vi "DataLogging.vi"() -> ()   [LabVIEW 2016]
uses:
  <vilib>/Utility/file.llb/Write Delimited Spreadsheet (string).vi
  <vilib>/Utility/file.llb/Write Delimited Spreadsheet (DBL).vi
panel:
  out "Elapsed Time":dbl
  in  "stop":bool
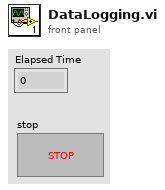
[diagram p1: front panel]
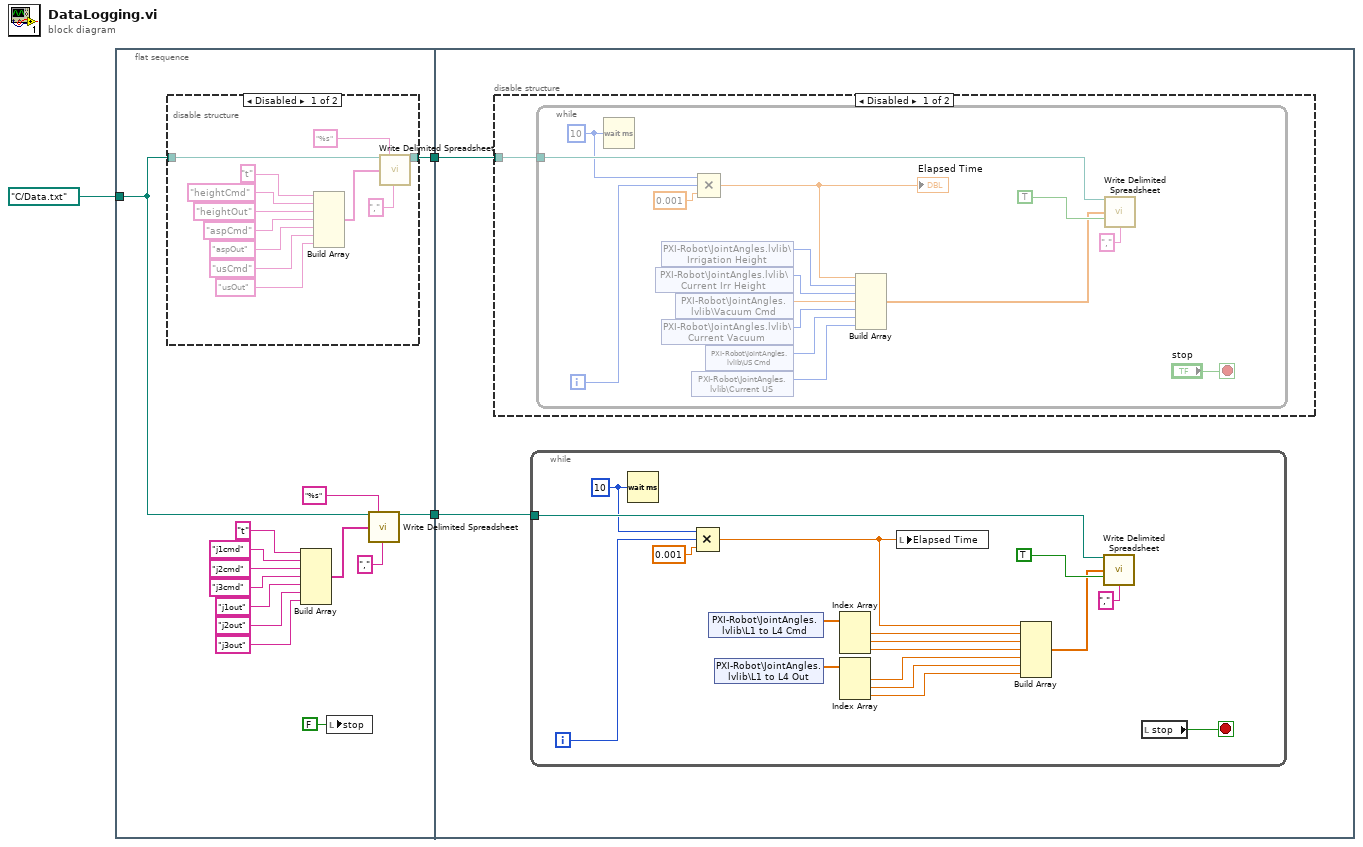
[diagram p0: block diagram]
diagram:
  n1 = flat-sequence {
    tunnel: [w17] -> w3
    tunnel: path "C:/Data.txt" ("Path") -> [w13]
    tunnel: [w5] -> w1
    tunnel: w3 -> [w31]
    tunnel: w1 -> [w30]
    frame #0 {
      n2 = disable-structure shown="Disabled" {
        disable-tunnel: [w20 _] -> w17
        disable-tunnel: w13 -> [w18 _]
        frame Disabled {
          n3 = Build Array("t" ("delimiter (\\t)"), "heightCmd" ("delimiter (\\t)"), "heightOut" ("delimiter (\\t)"), "aspCmd" ("delimiter (\\t)"), "aspOut" ("delimiter (\\t)"), "usCmd" ("delimiter (\\t)"), "usOut" ("delimiter (\\t)")) -> (w22:string[])
          n4 = call-poly <vilib>:"Write Delimited Spreadsheet.vi"("file path (dialog if empty)"=w18, "format (%s)"="%s", "1D data"=w22, "delimiter (\\t)"="," ("delimiter (\\t)")) -> ("new file path (Not A Path if cancelled)"=w20:path)  [unwired: 10 in, 1 out]
        }
        frame Enabled {
        }
      }
      n5 = Build Array("t" ("delimiter (\\t)"), "j1cmd" ("delimiter (\\t)"), "j2cmd" ("delimiter (\\t)"), "j3cmd" ("delimiter (\\t)"), "j1out" ("delimiter (\\t)"), "j2out" ("delimiter (\\t)"), "j3out" ("delimiter (\\t)")) -> (w14:string[])
      n6 = local write "stop"(FALSE ("stop")) -> ()
      n7 = call-poly <vilib>:"Write Delimited Spreadsheet.vi"("file path (dialog if empty)"=w13, "format (%s)"="%s", "1D data"=w14, "delimiter (\\t)"="," ("delimiter (\\t)")) -> ("new file path (Not A Path if cancelled)"=w5:path)  [unwired: 10 in, 1 out]
    }
    frame #1 {
      n8 = disable-structure shown="Disabled" {
        disable-tunnel: w31 -> [w49 _]
        frame Disabled {
          n9 = while {
            tunnel: w49 -> [w62]
            i -> [w52]
            stop <- "stop" stop-if-true
            w51 = u32 10 ("milliseconds to wait")
            n10 = Wait (ms)(milliseconds to wait=w51) -> ()  [unwired: 1 out]
            n11 = shared-variable "PXI-Robot\\JointAngles.lvlib\\Current Irr Height"() -> (w55:i32)  [unwired: 1 in, 1 out]
            n12 = shared-variable "PXI-Robot\\JointAngles.lvlib\\Irrigation Height"() -> (w54:i32)  [unwired: 1 in, 1 out]
            n13 = shared-variable "PXI-Robot\\JointAngles.lvlib\\Current Vacuum"() -> (w57:i32)  [unwired: 1 in, 1 out]
            n14 = shared-variable "PXI-Robot\\JointAngles.lvlib\\Vacuum Cmd"() -> (w56:sgl)  [unwired: 1 in, 1 out]
            n15 = shared-variable "PXI-Robot\\JointAngles.lvlib\\Current US"() -> (w59:i32)  [unwired: 1 in, 1 out]
            n16 = Compound Arithmetic op=MULTIPLY(w51, w52, 0.001 ("y")) -> (w50:dbl)
            "Elapsed Time" <- w50
            n17 = shared-variable "PXI-Robot\\JointAngles.lvlib\\US Cmd"() -> (w58:i32)  [unwired: 1 in, 1 out]
            n18 = Build Array(w50, w54, w55, w56, w57, w58, w59) -> (w61:dbl[])
            n19 = call-poly <vilib>:"Write Delimited Spreadsheet.vi"("file path (dialog if empty)"=w62, "1D data"=w61, "append to file? (new file:F)"=TRUE, "delimiter (\\t)"="," ("delimiter (\\t)")) -> ()  [unwired: 10 in, 2 out]
          }
        }
        frame Enabled {
        }
      }
      n20 = while {
        tunnel: w30 -> [w46]
        i -> [w43]
        stop <- w41 stop-if-true
        w40 = u32 10 ("milliseconds to wait")
        n21 = Wait (ms)(milliseconds to wait=w40) -> ()  [unwired: 1 out]
        n22 = Compound Arithmetic op=MULTIPLY(w40, w43, 0.001 ("y")) -> (w42:dbl)
        n23 = shared-variable "PXI-Robot\\JointAngles.lvlib\\L1 to L4 Cmd"() -> (w39:dbl[])  [unwired: 1 in, 1 out]
        n24 = shared-variable "PXI-Robot\\JointAngles.lvlib\\L1 to L4 Out"() -> (w35:dbl[])  [unwired: 1 in, 1 out]
        n25 = Index Array(array=w39) -> (element #1=w38:dbl, element #2=w37:dbl, element #3=w36:dbl)  [unwired: 3 in]
        n26 = Index Array(array=w35) -> (element #1=w34:dbl, element #2=w33:dbl, element #3=w32:dbl)  [unwired: 3 in]
        n27 = local write "Elapsed Time"(w42) -> ()
        n28 = Build Array(w42, w38, w37, w36, w34, w33, w32) -> (w45:dbl[])
        n29 = call-poly <vilib>:"Write Delimited Spreadsheet.vi"("file path (dialog if empty)"=w46, "1D data"=w45, "append to file? (new file:F)"=TRUE, "delimiter (\\t)"="," ("delimiter (\\t)")) -> ()  [unwired: 10 in, 2 out]
        n30 = local read "stop"() -> (w41:bool)
      }
    }
  }
